vi "SF2_Hault.vi"   [LabVIEW 2016]
uses:
  _Notifier/SF2_ActionTypeDef.ctl
types:
  T1 = typedef "SF2_ActionTypeDef.ctl" = enum16{"None", "Halt", "Reset Buffer"}
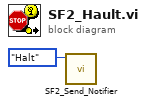
[diagram p0: block diagram]
diagram:
  n1 = call "SF2_Send_Notifier.vi"("SF2 Action"=SF2_ActionTypeDef."Halt") -> ()  [unwired: 11 in]
